vi "Parse Status Header.vi"(7 "Status Header In":string, 11 "error in (no error)":errorcluster) -> (1 "Full Spectrum Starting Wavelength (nm)":dbl, 2 "Full Spectrum Ending Wavelength (nm)":dbl, 3 "Granularity":u32, 6 "Number of Sensors":u16[](array[numeric]), 8 "Status":T2 {"Time Stamp" format="%#_20f"; "Operating Mode" items=["Stand-Alone", "Master", "End Slave", "Middle Slave"]; "Trigger Mode" items=["Untriggered", "Software Triggered", "Hardware Triggered"]}, 10 "Reserved":T1, 15 "error out":errorcluster)   [LabVIEW 2015, in "Micron Optics sm130.lvlib"]
doc: "Parses the status header that is included in every data retrieval."
uses:
  Micron Optics sm130.lvlib
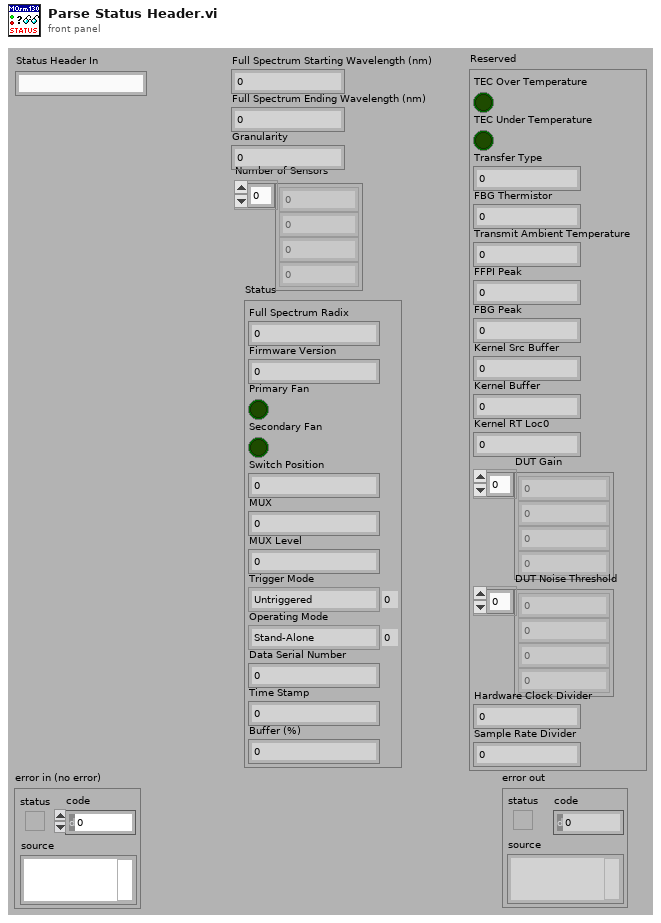
[diagram p1: front panel]
types:
  T1 = cluster{"Transmit Ambient Temperature":dbl, "FBG Thermistor":i16, "FFPI Peak":u16, "FBG Peak":dbl, "Kernel Src Buffer":u16, "Kernel Buffer":u16, "Kernel RT Loc0":u32, "DUT Gain":u16[], "DUT Noise Threshold":u16[], "Hardware Clock Divider":u16, "Sample Rate Divider":u16, "TEC Over Temperature":bool, "TEC Under Temperature":bool, "Transfer Type":u8}
  T2 = cluster{"Full Spectrum Radix":u8, "Firmware Version":u8, "Primary Fan":bool, "Secondary Fan":bool, "Switch Position":u8, "MUX":u8, "Trigger Mode":u8, "Operating Mode":u8, "Data Serial Number":u32, "Time Stamp":dbl, "Buffer (%)":u8, "MUX Level":u8}
  T3 = cluster{"Transmit Ambient Temperature":dbl, "FBG Thermistor":i16, "FFPI Peaks":u16, "FBG Peaks":dbl, "Kernel Src Buffer":u16, "Kernel Buffer":u16, "Kernel RT Loc0":u32, "DUT Gain":u16[], "DUT Noise Threshold":u16[], "Hardware Clock Divider":u16, "Peaks Data Rate Divider":u16, "TEC Over Temperature":bool, "TEC Under Temperature":bool, "Transfer Type":u8}
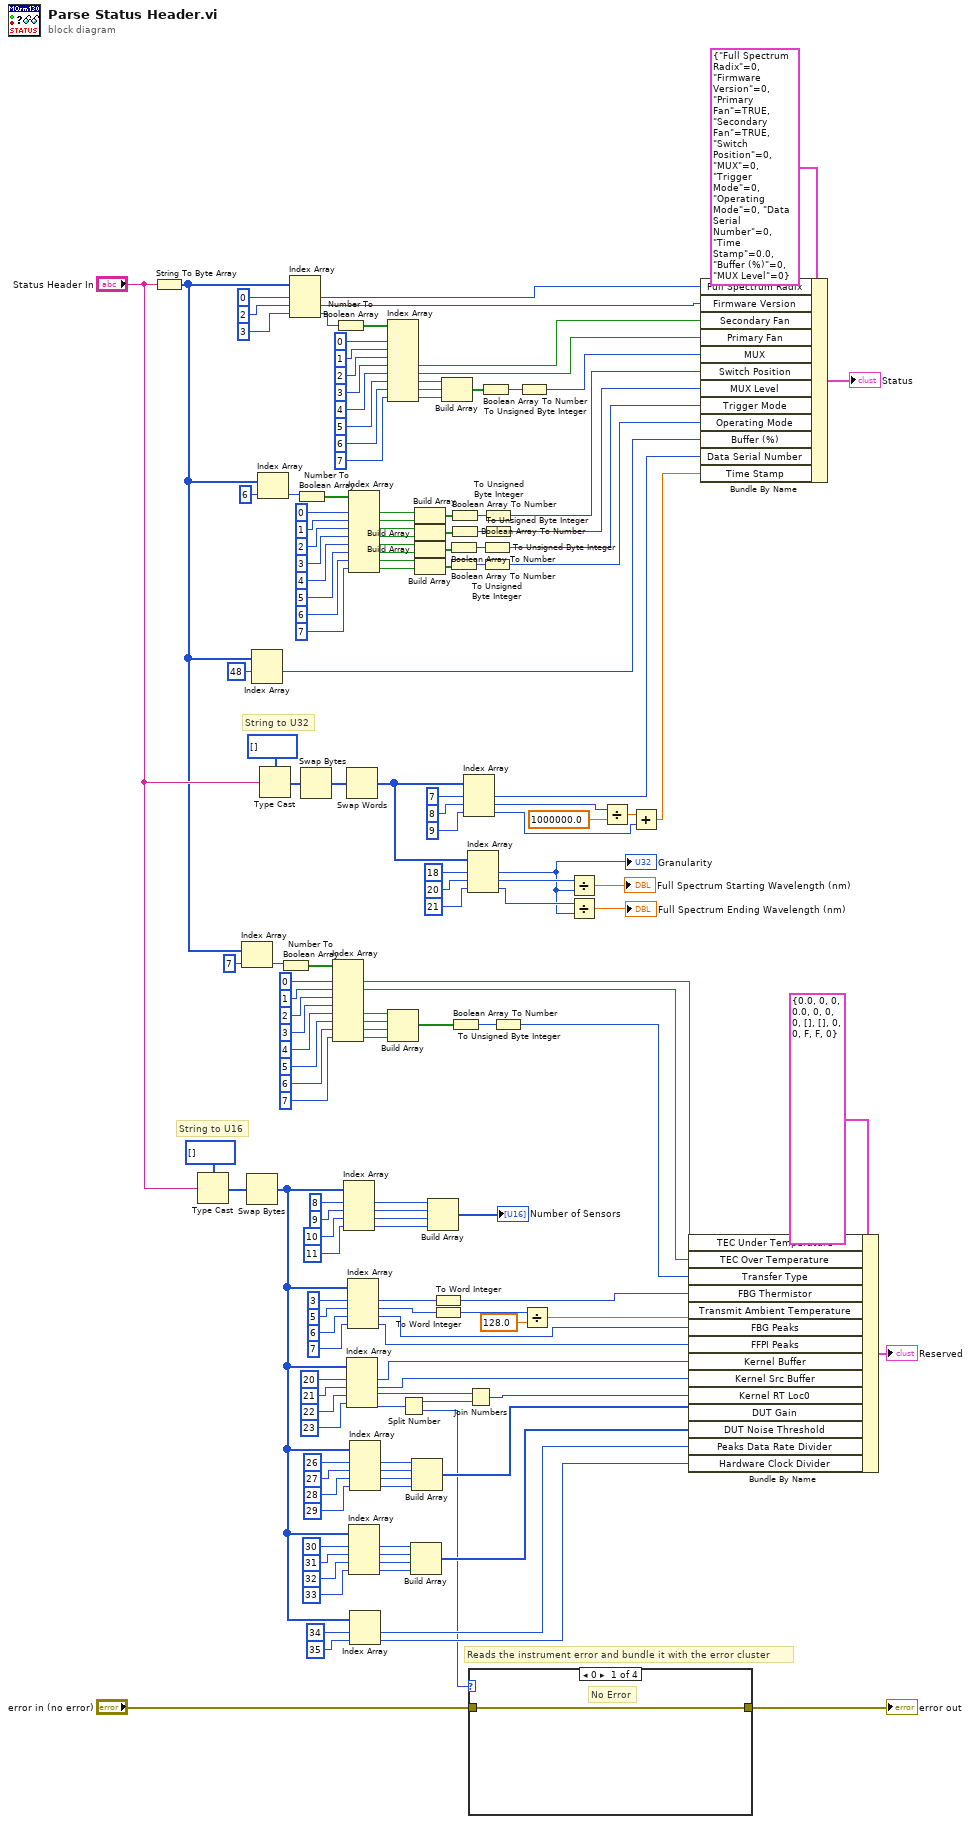
[diagram p0: block diagram]
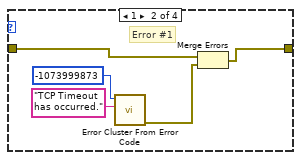
[diagram p2: hidden frame]
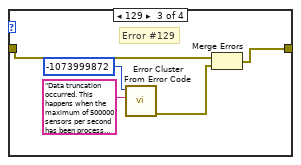
[diagram p3: hidden frame]
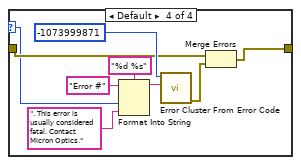
[diagram p4: hidden frame]
diagram:
  # "Reads the instrument error and bundle it with the error cluster"
  # "String to U16"
  # "String to U32"
  n1 = String To Byte Array(string="Status Header In") -> (unsigned byte array=w20:u8[])
  n2 = Type Cast(type=u16[] [], x="Status Header In") -> (*(type *) &x=w110:u16[])
  n3 = Index Array(array=w20, index=7) -> (element=w21:u8)
  n4 = Swap Bytes(anything=w110) -> (byte swapped=w61:u16[])
  n5 = Index Array(array=w20, index #1=48 ("index")) -> (element #1=w55:u8)  [unwired: 1 in, 1 out]
  n6 = Index Array(array=w20, index=6) -> (element=w127:u8)
  n7 = Type Cast(type=u32[] [], x="Status Header In") -> (*(type *) &x=w54:u32[])
  n8 = Number To Boolean Array(number=w21) -> (Boolean array=w30:bool[])
  n9 = Index Array(array=w20, index #1=0 ("index"), index #2=2 ("index"), index #3=3 ("index")) -> (element #1=w158:u8, element #2=w157:u8, element #3=w156:u8)
  n10 = Number To Boolean Array(number=w127) -> (Boolean array=w136:bool[])
  n11 = Swap Bytes(anything=w54) -> (byte swapped=w52:u32[])
  n12 = Index Array(array=w30, index #1=0 ("index"), index #2=1 ("index"), index #3=2 ("index"), index #4=3 ("index"), index #5=4 ("index"), index #6=5 ("index"), index #7=6 ("index"), index #8=7 ("index")) -> (element #1=w19:bool, element #2=w18:bool, element #5=w17:bool, element #6=w16:bool, element #7=w15:bool, element #8=w14:bool)  [unwired: 2 out]
  n13 = Number To Boolean Array(number=w156) -> (Boolean array=w155:bool[])
  n14 = Index Array(array=w61, index #1=8 ("index"), index #2=9 ("index"), index #3=10 ("index"), index #4=11 ("index")) -> (element #1=w105:u16, element #2=w104:u16, element #3=w103:u16, element #4=w102:u16)
  n15 = Swap Words(1:w52) -> (0:w38:u32[])
  n16 = Index Array(array=w61, index #1=20 ("index"), index #2=21 ("index"), index #3=22 ("index"), index #4=23 ("index")) -> (element #1=w85:u16, element #2=w84:u16, element #3=w81:u16, element #4=w83:u16)
  n17 = Index Array(array=w61, index #1=3 ("index"), index #2=5 ("index"), index #3=6 ("index"), index #4=7 ("index")) -> (element #1=w100:u16, element #2=w97:u16, element #3=w92:u16, element #4=w90:u16)
  n18 = Index Array(array=w136, index #1=0 ("index"), index #2=1 ("index"), index #3=2 ("index"), index #4=3 ("index"), index #5=4 ("index"), index #6=5 ("index"), index #7=6 ("index"), index #8=7 ("index")) -> (element #1=w126:bool, element #2=w125:bool, element #3=w6:bool, element #4=w5:bool, element #5=w119:bool, element #6=w118:bool, element #7=w115:bool, element #8=w114:bool)
  n19 = Index Array(array=w61, index #1=30 ("index"), index #2=31 ("index"), index #3=32 ("index"), index #4=33 ("index")) -> (element #1=w68:u16, element #2=w67:u16, element #3=w69:u16, element #4=w70:u16)
  n20 = Index Array(array=w61, index #1=26 ("index"), index #2=27 ("index"), index #3=28 ("index"), index #4=29 ("index")) -> (element #1=w74:u16, element #2=w75:u16, element #3=w73:u16, element #4=w72:u16)
  n21 = Index Array(array=w61, index #1=34 ("index"), index #2=35 ("index")) -> (element #1=w58:u16, element #2=w57:u16)
  n22 = Index Array(array=w155, index #1=0 ("index"), index #2=1 ("index"), index #3=2 ("index"), index #4=3 ("index"), index #5=4 ("index"), index #6=5 ("index"), index #7=6 ("index"), index #8=7 ("index")) -> (element #4=w146:bool, element #5=w145:bool, element #6=w143:bool, element #7=w142:bool, element #8=w141:bool)  [unwired: 3 out]
  n23 = Build Array(w17, w16, w15, w14) -> (w13:bool[])
  n24 = Split Number(x=w83) -> (hi(x)=w82:u8, lo(x)=w3:u8)
  n25 = Build Array(w68, w67, w69, w70) -> (w62:u16[])
  n26 = Build Array(w74, w75, w73, w72) -> (w71:u16[])
  n27 = Build Array(w126, w125) -> (w123:bool[])
  n28 = Build Array(w6, w5) -> (w8:bool[])
  n29 = Build Array(w119, w118) -> (w121:bool[])
  n30 = Build Array(w115, w114) -> (w116:bool[])
  n31 = Build Array(w105, w104, w103, w102) -> (→"Number of Sensors":u16[])
  n32 = To Word Integer(number=w100) -> (16bit integer=w99:i16)
  n33 = To Word Integer(number=w97) -> (16bit integer=w95:i16)
  n34 = Build Array(w143, w142, w141) -> (w144:bool[])
  n35 = Boolean Array To Number(Boolean array=w121) -> (number=w120:u32)
  n36 = Boolean Array To Number(Boolean array=w116) -> (number=w117:u32)
  n37 = Boolean Array To Number(Boolean array=w123) -> (number=w124:u32)
  n38 = Boolean Array To Number(Boolean array=w8) -> (number=w7:u32)
  n39 = Boolean Array To Number(Boolean array=w13) -> (number=w12:u32)
  n40 = Index Array(array=w38, index #1=7 ("index"), index #2=8 ("index"), index #3=9 ("index")) -> (element #1=w49:u32, element #2=w44:u32, element #3=w43:u32)
  n41 = Join Numbers(hi=w81, lo=w82) -> ((hi.lo)=w80:u32)
  n42 = Index Array(array=w38, index #1=18 ("index"), index #2=20 ("index"), index #3=21 ("index")) -> (element #1=w35:u32, element #2=w37:u32, element #3=w36:u32)
  "Granularity" <- w35
  n43 = case shown="0" w3 {
    selector: w3 -> [_ _ _ w178]
    tunnel: "error in (no error)" -> [w163 w164 w170 w180]
    tunnel: [w163 w166 w169 w179] -> w1
    frame 0 {
      # "No Error"
    }
    frame 1 {
      # "Error #1"
      n44 = call <vilib>:"Error Cluster From Error Code.vi"("error message (\"\")"="TCP Timeout has occurred." ("error message (\"\")"), "error code (0)"=-1073999873) -> ("error out"=w165:errorcluster)  [unwired: 7 in]
      n45 = Merge Errors(w164, w165) -> (w166:errorcluster)
    }
    frame 129 {
      # "Error #129"
      n46 = call <vilib>:"Error Cluster From Error Code.vi"("error message (\"\")"="Data truncation occurred. This happens when the maximum of 500000 sensors per second has been processed." ("error message (\"\")"), "error code (0)"=-1073999872) -> ("error out"=w171:errorcluster)  [unwired: 7 in]
      n47 = Merge Errors(w170, w171) -> (w169:errorcluster)
    }
    frame Default {
      n48 = Format Into String(format string="%d %s", initial string="Error #", w178, ". This error is usually considered fatal. Contact Micron Optics." ("error message (\"\")")) -> (resulting string=w177:string)  [unwired: 1 in, 1 out]
      n49 = call <vilib>:"Error Cluster From Error Code.vi"("error message (\"\")"=w177, "error code (0)"=-1073999871) -> ("error out"=w181:errorcluster)  [unwired: 7 in]
      n50 = Merge Errors(w180, w181) -> (w179:errorcluster)
    }
  }
  "error out" <- w1
  n51 = Boolean Array To Number(Boolean array=w144) -> (number=w140:u32)
  n52 = To Unsigned Byte Integer(number=w120) -> (unsigned 8bit integer=w10:u8)
  n53 = To Unsigned Byte Integer(number=w117) -> (unsigned 8bit integer=w113:u8)
  n54 = To Unsigned Byte Integer(number=w124) -> (unsigned 8bit integer=w122:u8)
  n55 = To Unsigned Byte Integer(number=w7) -> (unsigned 8bit integer=w4:u8)
  n56 = To Unsigned Byte Integer(number=w12) -> (unsigned 8bit integer=w11:u8)
  n57 = To Unsigned Byte Integer(number=w140) -> (unsigned 8bit integer=w139:u8)
  n58 = Divide(x=w95, y=128.0) -> (x/y=w94:dbl)
  n59 = Divide(x=w37, y=w35) -> (x/y=→"Full Spectrum Starting Wavelength (nm)":dbl)
  n60 = Divide(x=w36, y=w35) -> (x/y=→"Full Spectrum Ending Wavelength (nm)":dbl)
  n61 = Divide(x=w44, y=1000000.0) -> (x/y=w45:dbl)
  n62 = Add(x=w45, y=w43) -> (x+y=w42:dbl)
  n63 = Bundle By Name(cluster=T3 {"Transmit Ambient Temperature"=0.0, "FBG Thermistor"=0, "FFPI Peaks"=0, "FBG Peaks"=0.0, "Kernel Src Buffer"=0, "Kernel Buffer"=0, "Kernel RT Loc0"=0, "DUT Gain"=[], "DUT Noise Threshold"=[], "Hardware Clock Divider"=0, "Peaks Data Rate Divider"=0, "TEC Over Temperature"=FALSE, "TEC Under Temperature"=FALSE, "Transfer Type"=0} ("Reserved 2"), "TEC Under Temperature"=w19, "TEC Over Temperature"=w18, "Transfer Type"=w11, "FBG Thermistor"=w99, "Transmit Ambient Temperature"=w94, "FBG Peaks"=w92, "FFPI Peaks"=w90, "Kernel Buffer"=w85, "Kernel Src Buffer"=w84, "Kernel RT Loc0"=w80, "DUT Gain"=w71, "DUT Noise Threshold"=w62, "Peaks Data Rate Divider"=w58, "Hardware Clock Divider"=w57) -> (→"Reserved":T3)
  n64 = Bundle By Name(cluster=T2 {"Full Spectrum Radix"=0, "Firmware Version"=0, "Primary Fan"=TRUE, "Secondary Fan"=TRUE, "Switch Position"=0, "MUX"=0, "Trigger Mode"=0, "Operating Mode"=0, "Data Serial Number"=0, "Time Stamp"=0.0, "Buffer (%)"=0, "MUX Level"=0} ("Status 2"), "Full Spectrum Radix"=w158, "Firmware Version"=w157, "Secondary Fan"=w146, "Primary Fan"=w145, "MUX"=w139, "Switch Position"=w122, "MUX Level"=w4, "Trigger Mode"=w10, "Operating Mode"=w113, "Buffer (%)"=w55, "Data Serial Number"=w49, "Time Stamp"=w42) -> (→"Status":T2)
